vi "Call protocol STOP on error.vi"(8 "error in (no error)":errorcluster) -> (0 "error out":errorcluster)   [LabVIEW 2017]
uses:
  Typedefs/Top level VI states.ctl
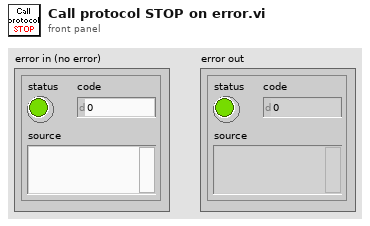
[diagram p1: front panel]
types:
  T1 = typedef "Imaging Protocols enum.ctl" = enum16{"AOL Z-Stack", "Motor Z Stack", "Parameter Sweep", "Functional Acquisition", "Single Plane Acquisition", "Volume Acquisition", "Live Imaging", "Live Plane Imaging", "Live Volume Imaging"}
  T2 = typedef "Top level VI states.ctl" = enum16{"None", "Initialise UI", "<STACK PROTOCOL STATES>", "AOL Zstack-START", "AOL Zstack-STOP", "Motor Zstack-START", "Motor Zstack-STOP", "Parameter Sweep-START", "Parameter Sweep-STOP", "<ACQUISITION PROTOCOL STATES> ", "Functional Acquisition-START", "Functional Acquisition-STOP", "Single Plane Acquisition-START", "Single Plane Acquisition-STOP", "Volume Acquisition-START", "Volume Acquisition-STOP", "<LIVE IMAGING PROTOCOL STATES>", "Live Imaging-START", "Live Imaging-STOP", "Live Plane Imaging-START", "Live Plane Imaging-STOP", "Live Volume Imaging-START", "Live Volume Imaging-STOP", "<MOVEMENT CORRECTION PROTOCOL STATES>", "EXIT"}
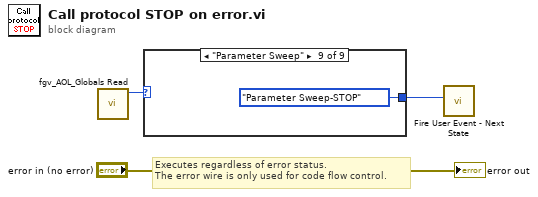
[diagram p0: block diagram]
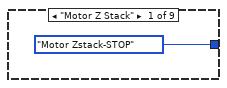
[diagram p2: hidden frame]
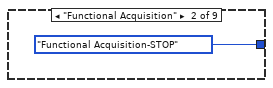
[diagram p3: hidden frame]
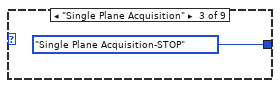
[diagram p4: hidden frame]
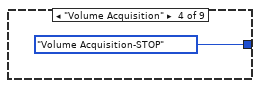
[diagram p5: hidden frame]
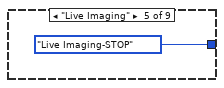
[diagram p6: hidden frame]
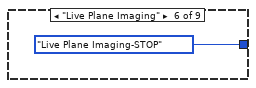
[diagram p7: hidden frame]
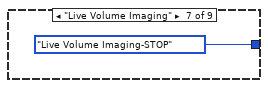
[diagram p8: hidden frame]
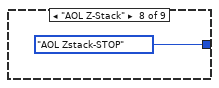
[diagram p9: hidden frame]
diagram:
  # "Executes regardless of error status.\nThe error wire is only used for code flow control."
  n1 = call "fgv_AOL_Globals Read.vi"() -> ("Imaging Protocol"=w1:T1)  [unwired: 9 in, 2 out]
  n2 = case shown="\"Parameter Sweep\"" w1 {
    tunnel: [Top_level_VI_states."Motor Zstack-STOP" ("event data / imaging mode") Top_level_VI_states."Functional Acquisition-STOP" ("event data / imaging mode") Top_level_VI_states."Single Plane Acquisition-STOP" ("event data / imaging mode") Top_level_VI_states."Volume Acquisition-STOP" ("event data / imaging mode") Top_level_VI_states."Live Imaging-STOP" ("event data / imaging mode") Top_level_VI_states."Live Plane Imaging-STOP" ("event data / imaging mode") Top_level_VI_states."Live Volume Imaging-STOP" ("event data / imaging mode") Top_level_VI_states."AOL Zstack-STOP" ("event data / imaging mode") Top_level_VI_states."Parameter Sweep-STOP" ("event data / imaging mode")] -> w2
    frame "Motor Z Stack" {
    }
    frame "Functional Acquisition" {
    }
    frame "Single Plane Acquisition" {
    }
    frame "Volume Acquisition" {
    }
    frame "Live Imaging" {
    }
    frame "Live Plane Imaging" {
    }
    frame "Live Volume Imaging" {
    }
    frame "AOL Z-Stack" {
    }
    frame "Parameter Sweep" {
    }
  }
  n3 = call "Fire User Event - Next State.vi"("\"UI Handler loop\" case to execute"=w2) -> ()  [unwired: 10 in, 1 out]
  "error out" <- "error in (no error)"
